vi "DAQ_A&D_tb.vi"() -> ()   [LabVIEW 2018]
panel:
  out "Digital Waveform Graph 3":digitalwaveform[](graph)
  out "Digital Waveform Graph 2":digitalwaveform[](graph)
  out "Digital Waveform Graph":digitalwaveform[](graph)
  in  "stop":bool
  out "Waveform Graph 3":dynamicdata(graph)
  out "Waveform Graph 2":dynamicdata(graph)
  out "Waveform Graph":dynamicdata(graph)
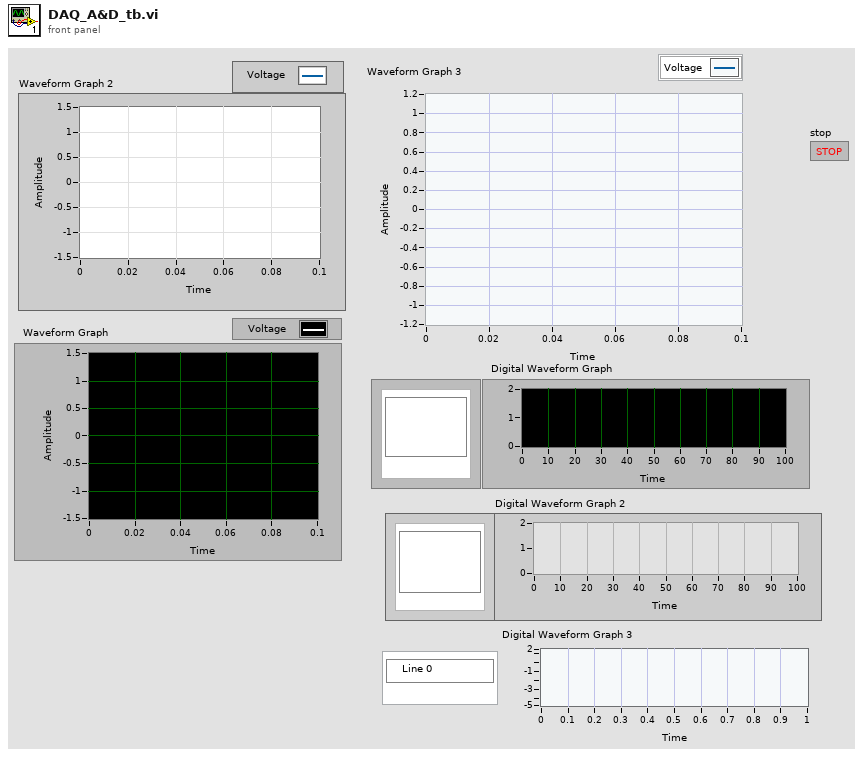
[diagram p1: front panel]
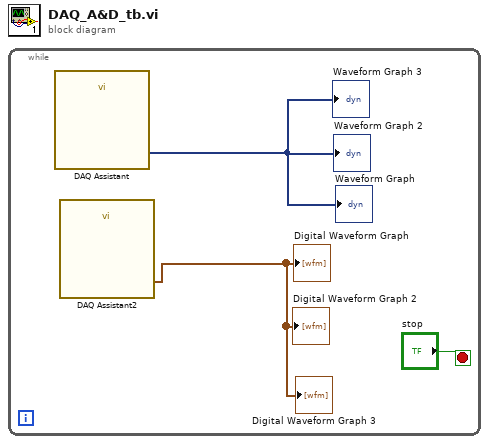
[diagram p0: block diagram]
diagram:
  n1 = while {
    stop <- "stop" stop-if-true
    n2 = call "DAQ Assistant"() -> ("data"=→"Waveform Graph" →"Waveform Graph 2" →"Waveform Graph 3":dynamicdata)  [unwired: 17 in, 2 out]
    n3 = call "DAQ Assistant2"() -> ("data"=→"Digital Waveform Graph" →"Digital Waveform Graph 2" →"Digital Waveform Graph 3":digitalwaveform[])  [unwired: 17 in, 2 out]
  }
